vi "stop.vi"(8 "error in (no error)":errorcluster, 10 "stop?":bool, 11 "SpinCore in":refnum<class "SpinCore.lvclass">) -> (0 "error out":errorcluster, 2 "hasStopped":bool, 3 "SpinCore out":refnum<class "SpinCore.lvclass">)   [LabVIEW 2011, in "Hardware.lvlib" / "Channels.lvlib" / "SpinCore.lvclass"]
uses:
  SpinCore.lvclass
  SpinCore.lvclass/SpinCore.ctl
panel:
  out "Boolean array":bool[](array[boolean])
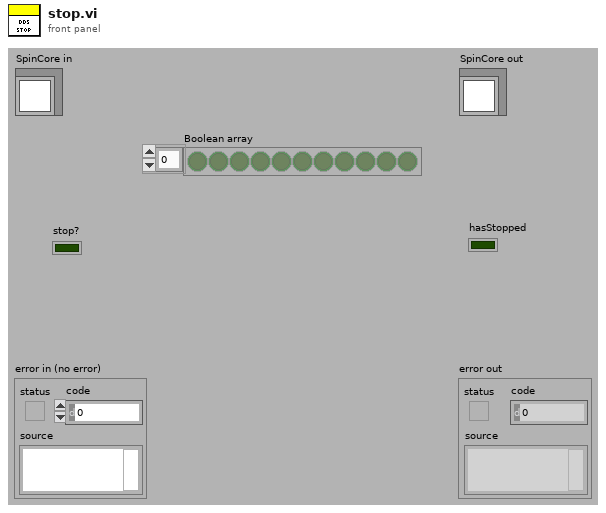
[diagram p1: front panel]
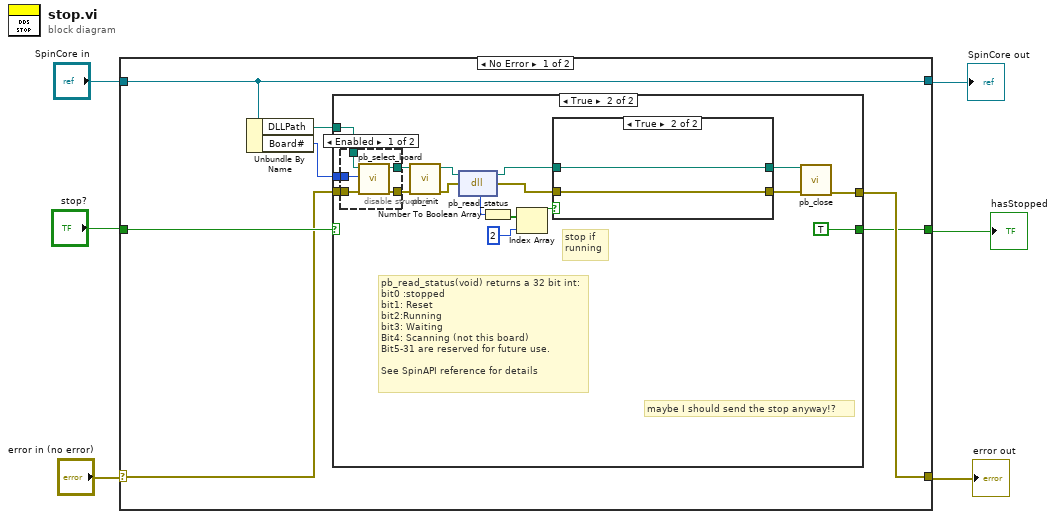
[diagram p0: block diagram]
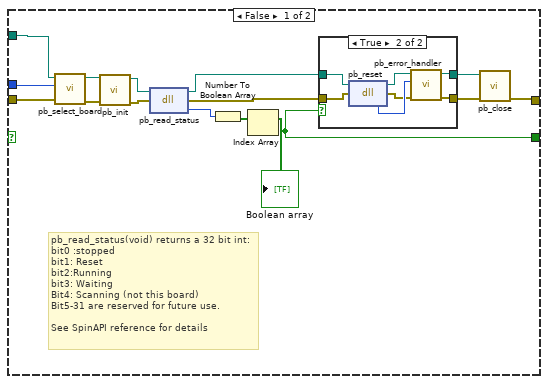
[diagram p2: hidden frame]
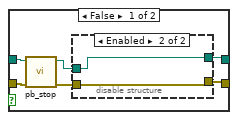
[diagram p5: hidden frame]
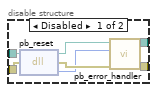
[diagram p6: hidden frame]
diagram:
  n1 = case shown="No Error" "error in (no error)" {
    selector: "error in (no error)" -> [w9 w79]
    tunnel: [w8 w79] -> w5
    tunnel: [w13 w80] -> w4
    tunnel: "SpinCore in" -> [w13 w80]
    tunnel: "stop?" -> [w12 _]
    tunnel: [w7 _] -> w1
    frame No Error {
      n2 = Unbundle By Name(w13) -> ("DLLPath"=w11:path, "Board#"=w10:i32)
      n3 = case shown="True" w12 {
        tunnel: w11 -> [w25 w50]
        tunnel: w10 -> [w26 w49]
        tunnel: w9 -> [w28 w48]
        tunnel: [w27 w47] -> w8
        tunnel: [w18 TRUE] -> w7
        frame False {
          # "pb_read_status(void) returns a 32 bit int:\nbit0 :stopped\nbit1: Reset\nbit2:Running\nbit3: Waiting\nBit4: Scanning (not this board)\nBit5-31 are reserved for future use.\n\nSee SpinAPI reference for details"
          n4 = call <userlib>:"pb_select_board.vi"("error in (no error)"=w28, "board_num"=w26, "path in"=w25) -> ("error out"=w24:errorcluster, "path out"=w23:path)  [unwired: 7 in]
          n5 = call <userlib>:"pb_init.vi"("error in (no error)"=w24, "path in"=w23) -> ("error out"=w22:errorcluster, "path out"=w19:path)  [unwired: 8 in]
          n6 = dll-call lib="C:/Program Files/National Instruments/LabVIEW 2009/spinapi.dll" fn="pb_read_status"(path in=w19, error in=w22) -> (path out=w17:path, error out=w15:errorcluster, "status"=w21:i32)  [unwired: 1 in]
          n7 = Number To Boolean Array(number=w21) -> (Boolean array=w20:bool[])
          "Boolean array" <- w20
          n8 = Index Array(array=w20) -> (element=w18:bool)  [unwired: 1 in]
          n9 = case shown="True" w18 {
            tunnel: w17 -> [w30 w37]
            tunnel: [w30 w35] -> w16
            tunnel: w15 -> [w29 w36]
            tunnel: [w29 w34] -> w14
            frame False {
            }
            frame True {
              n10 = dll-call lib="C:/Program Files/National Instruments/LabVIEW 2009/spinapi.dll" fn="pb_reset"(path in=w37, error in=w36) -> (path out=w32:path, error out=w31:errorcluster, "error"=w33:i32)  [unwired: 1 in]
              n11 = call <userlib>:"pb_error_handler.vi"("error in (no error)"=w31, "return code"=w33, "path in"=w32) -> ("error out"=w34:errorcluster, "path out"=w35:path)  [unwired: 7 in]
            }
          }
          n12 = call <userlib>:"pb_close.vi"("error in (no error)"=w14, "path in"=w16) -> ("error out"=w27:errorcluster)  [unwired: 8 in, 1 out]
        }
        frame True {
          # "maybe I should send the stop anyway!?"
          # "stop if \nrunning"
          # "pb_read_status(void) returns a 32 bit int:\nbit0 :stopped\nbit1: Reset\nbit2:Running\nbit3: Waiting\nBit4: Scanning (not this board)\nBit5-31 are reserved for future use.\n\nSee SpinAPI reference for details"
          n13 = disable-structure shown="Enabled" {
            disable-tunnel: [w59 w60] -> w54
            disable-tunnel: [w58 w61] -> w53
            disable-tunnel: w50 -> [w57 w61]
            disable-tunnel: w49 -> [w56 _]
            disable-tunnel: w48 -> [w55 w60]
            frame Enabled {
              n14 = call <userlib>:"pb_select_board.vi"("error in (no error)"=w55, "board_num"=w56, "path in"=w57) -> ("error out"=w59:errorcluster, "path out"=w58:path)  [unwired: 7 in]
            }
            frame Disabled {
            }
          }
          n15 = call <userlib>:"pb_init.vi"("error in (no error)"=w54, "path in"=w53) -> ("error out"=w42:errorcluster, "path out"=w43:path)  [unwired: 8 in]
          n16 = dll-call lib="C:/Program Files/National Instruments/LabVIEW 2009/spinapi.dll" fn="pb_read_status"(path in=w43, error in=w42) -> (path out=w39:path, error out=w40:errorcluster, "status"=w45:i32)  [unwired: 1 in]
          n17 = Number To Boolean Array(number=w45) -> (Boolean array=w44:bool[])
          n18 = Index Array(array=w44, index=2) -> (element=w41:bool)
          n19 = case shown="True" w41 {
            tunnel: [w62 w77] -> w52
            tunnel: [w63 w78] -> w51
            tunnel: w40 -> [w67 w77]
            tunnel: w39 -> [w66 w78]
            frame False {
              n20 = call <userlib>:"pb_stop.vi"("error in (no error)"=w67, "path in"=w66) -> ("error out"=w64:errorcluster, "path out"=w65:path)  [unwired: 8 in]
              n21 = disable-structure shown="Enabled" {
                disable-tunnel: w65 -> [w74 w76]
                disable-tunnel: w64 -> [w73 w75]
                disable-tunnel: [w72 w76] -> w63
                disable-tunnel: [w71 w75] -> w62
                frame Disabled {
                  n22 = dll-call lib="C:/Program Files/National Instruments/LabVIEW 2009/spinapi.dll" fn="pb_reset"(path in=w74, error in=w73) -> (path out=w70:path, error out=w69:errorcluster, "error"=w68:i32)  [unwired: 1 in]
                  n23 = call <userlib>:"pb_error_handler.vi"("error in (no error)"=w69, "return code"=w68, "path in"=w70) -> ("error out"=w71:errorcluster, "path out"=w72:path)  [unwired: 7 in]
                }
                frame Enabled {
                }
              }
            }
            frame True {
            }
          }
          n24 = call <userlib>:"pb_close.vi"("error in (no error)"=w52, "path in"=w51) -> ("error out"=w47:errorcluster)  [unwired: 8 in, 1 out]
        }
      }
    }
    frame Error {
    }
  }
  "error out" <- w5
  "SpinCore out" <- w4
  "hasStopped" <- w1
